vi "Cinemática Inversa.vi"() -> ()   [LabVIEW 2013]
uses:
  <vilib>/imath/engines/lvmath2/RunTimeEngine/NodeEndStatement/NIMS_NodeEndStatement_Output.vi
  <instcachedir>/0/NIMS_NodeEndStatement_Output_53EC0D466D134D7ABD903AC30B43404B.lvgen/NIMS_NodeEndStatement_Output_53EC0D466D134D7ABD903AC30B43404B_009.vi
  <vilib>/imath/engines/lvmath2/RunTimeEngine/BuiltInFunctions/atan/NIMS_atan(C).vi
  <instcachedir>/0/NIMS_atan(C)_7C2C2596D2F04E9E823B85B74D765718.lvgen/NIMS_atan(C)_7C2C2596D2F04E9E823B85B74D765718_001.vi
  <vilib>/imath/engines/lvmath2/RunTimeEngine/ErrorHandling/NIMS_Finalize Error.vi
panel:
  out "MOTOR 3":dbl(knob) scale=-50.0..100.0
  out "MOTOR 2":dbl(knob) scale=-50.0..100.0
  out "MOTOR 1":dbl(knob) scale=-50.0..100.0
  in  "Z":dbl=-158.0 min=-320.0 max=-158.0
  in  "X":dbl min=-80.0 max=80.0
  in  "Y":dbl min=-80.0 max=80.0
  in  "STOP":bool
  # "VALORES EXTREMOS ORIENTATIVOS"
  # "Xmín =  - 80mm"
  # "Xmáx =  + 80mm"
  # "Ymín = - 80mm"
  # "Ymáx = + 80mm"
  # "Zmín  = - 320mm"
  # "Zmáx = - 158mm"
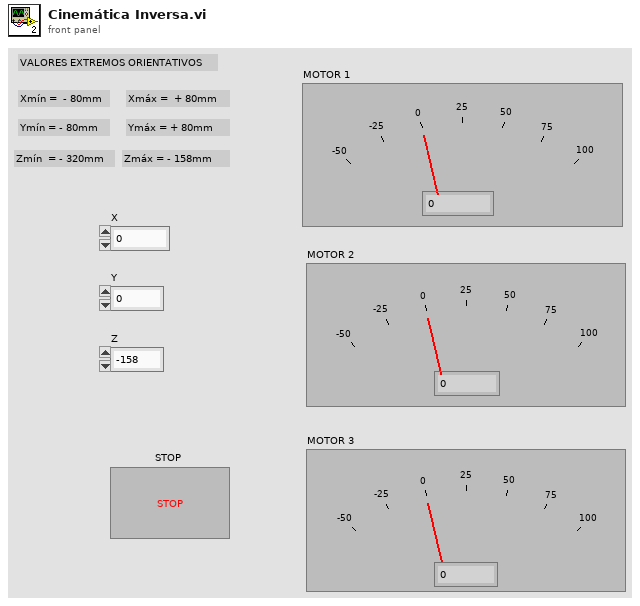
[diagram p1: front panel]
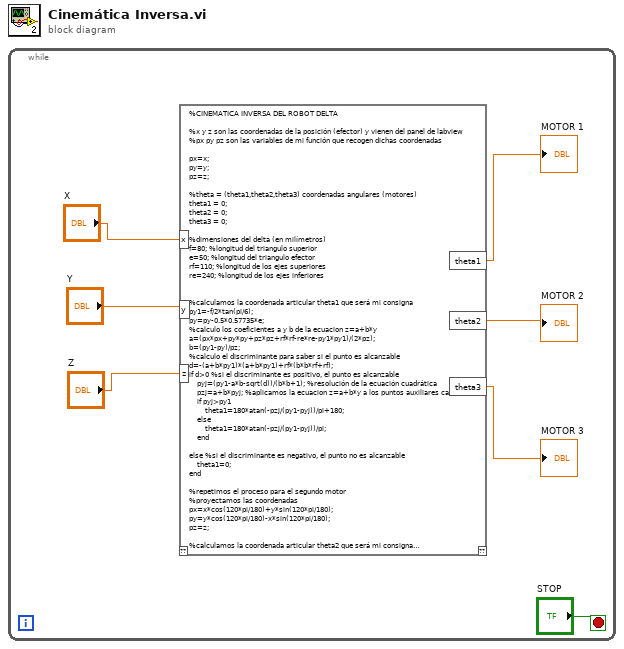
[diagram p0: block diagram]
diagram:
  n1 = while {
    stop <- "STOP" stop-if-true
    n2 = mathscript code="%CINEMATICA INVERSA DEL ROBOT DELTA\n\n%x y z son las coordenadas de la posición (efector) y vienen del panel de labview\n%px py pz son las variables de mi función que recogen dichas coordenadas\n\npx=x;\npy=y;\npz=z;\n\n%theta = (theta1,theta2,theta3) coordenadas angulares (motores)\ntheta1 = 0;\ntheta2 = 0;\ntheta3 = 0;\n\n%dimensiones del delta (en milímetros)\nf=80; %longitud del triangulo superior\ne=50; %longitud del triangulo efector\nrf=110; %longitud de los ejes superiores\nre=240; %longitud de los ejes inferiores\n\n\n%calculamos la coordenada articular theta1 que será mi consigna\npy1=-f/2*tan(pi/6);\npy=py-0.5*0.57735*e;\n%calculo los coeficientes a y b de la ecuacion z=a+b*y\na=(px*px+py*py+pz*pz+rf*rf-re*re-py1*py1)/(2*pz);\nb=(py1-py)/pz;\n%calculo el discriminante para saber si el punto es alcanzable\nd=-(a+b*py1)*(a+b*py1)+rf*(b*b*rf+rf);\nif d>0 %si el discriminante es positivo, el punto es alcanzable\n    pyj=(py1-a*b-sqrt(d))/(b*b+1); %resolución de la ecuación cuadrática\n    pzj=a+b*pyj; %aplicamos la ecuacion z=a+b*y a los puntos auxiliares calculados\n    if pyj>py1\n        theta1=180*atan(-pzj/(py1-pyj))/pi+180;\n    else\n        theta1=180*atan(-pzj/(py1-pyj))/pi;\n    end\n        \nelse %si el discriminante es negativo, el punto no es alcanzable\n    theta1=0;\nend\n\n%repetimos el proceso para el segundo motor\n%proyectamos las coordenadas\npx=x*cos(120*pi/180)+y*sin(120*pi/180);\npy=y*cos(120*pi/180)-x*sin(120*pi/180);\npz=z;\n\n%calculamos la coordenada articular theta2 que será mi consigna\npy1=-f/2*tan(pi/6);\npy=py-0.5*0.57735*e;\n%calculo los coeficientes a y b de la ecuacion z=a+b*y\na=(px*px+py*py+pz*pz+rf*rf-re*re-py1*py1)/(2*pz);\nb=(py1-py)/pz;\n%calculo el discriminante para saber si el punto es alcanzable\nd=-(a+b*py1)*(a+b*py1)+rf*(b*b*rf+rf);\nif d>0 %si el discriminante es positivo, el punto es alcanzable\n    pyj=(py1-a*b-sqrt(d))/(b*b+1); %resolución de la ecuación cuadrática\n    pzj=a+b*pyj; %aplicamos la ecuacion z=a+b*y a los puntos auxiliares calculados\n    if pyj>py1\n        theta2=180*atan(-pzj/(py1-pyj))/pi+180;\n    else\n        theta2=180*atan(-pzj/(py1-pyj))/pi;\n    end\n        \nelse %si el discriminante es negativo, el punto no es alcanzable\n    theta2=0;\nend\n\n%repetimos el proceso para el tercer motor\n%proyectamos las coordenadas\npx=x*cos(120*pi/180)-y*sin(120*pi/180);\npy=y*cos(120*pi/180)+x*sin(120*pi/180);\npz=z;\n\n%calculamos la coordenada articular theta3 que será mi consigna\npy1=-f/2*tan(pi/6);\npy=py-0.5*0.57735*e;\n%calculo los coeficientes a y b de la ecuacion z=a+b*y\na=(px*px+py*py+pz*pz+rf*rf-re*re-py1*py1)/(2*pz);\nb=(py1-py)/pz;\n%calculo el discriminante para saber si el punto es alcanzable\nd=-(a+b*py1)*(a+b*py1)+rf*(b*b*rf+rf);\nif d>0 %si el discriminante es positivo, el punto es alcanzable\n    pyj=(py1-a*b-sqrt(d))/(b*b+1); %resolución de la ecuación cuadrática\n    pzj=a+b*pyj; %aplicamos la ecuacion z=a+b*y a los puntos auxiliares calculados\n    if pyj>py1\n        theta3=180*atan(-pzj/(py1-pyj))/pi+180;\n    else\n        theta3=180*atan(-pzj/(py1-pyj))/pi;\n    end\n        \nelse %si el discriminante es negativo, el punto no es alcanzable\n    theta3=0;\nend\n\n%Ya tenemos nuestras coordenadas angulares para las x,y,z dadas\ntheta=[theta1,theta2,theta3];"("x"="X", "y"="Y", "z"="Z") -> ("theta1"=→"MOTOR 1":cdb, "theta2"=→"MOTOR 2":cdb, "theta3"=→"MOTOR 3":cdb)  [unwired: 1 in, 1 out]
  }
